vi "Check SUM.vi"() -> ()   [LabVIEW 2010, in "DCP551.lvlib"]
uses:
  DCP551.lvlib
panel:
  out "hex integer string 2":string
  out "Check Sum String":string
  in  "String Input":string
  out "*(type *) &x":string
  out "sum":u8 format="%04x"
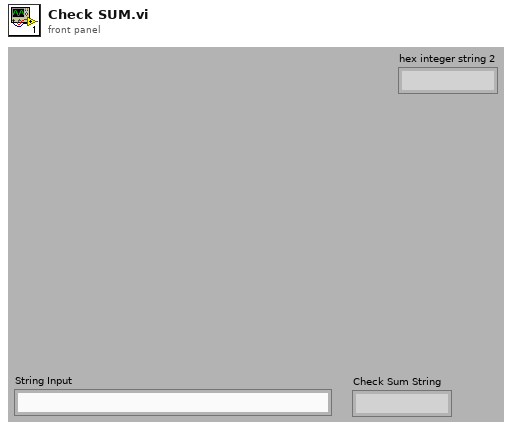
[diagram p1: front panel]
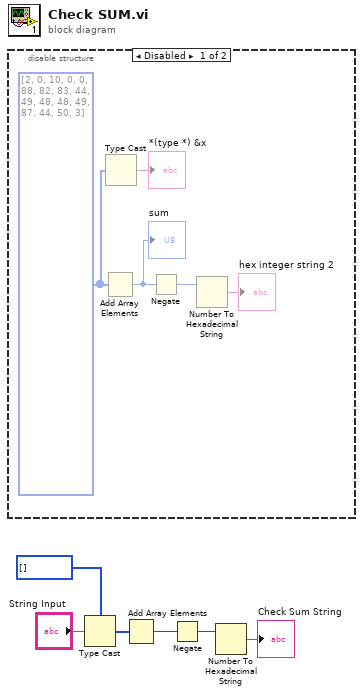
[diagram p0: block diagram]
diagram:
  n1 = disable-structure shown="Disabled" {
    frame Disabled {
      w11 = i8[] [2, 0, 10, 0, 0, 88, 82, 83, 44, 49, 48, 48, 49, 87, 44, 50, 3]
      n2 = Add Array Elements(numeric array=w11) -> (sum=w7:i8)
      "sum" <- w7
      n3 = Type Cast(x=w11) -> (*(type *) &x=→"*(type *) &x":string)  [unwired: 1 in]
      n4 = Negate(x=w7) -> (-x=w8:i8)
      n5 = Number To Hexadecimal String(2:w8) -> (0:→"hex integer string 2":string)  [unwired: 1 in]
    }
    frame Enabled {
    }
  }
  n6 = Type Cast(type=i8[] [], x="String Input") -> (*(type *) &x=w4:i8[])
  n7 = Add Array Elements(numeric array=w4) -> (sum=w3:i8)
  n8 = Negate(x=w3) -> (-x=w2:i8)
  n9 = Number To Hexadecimal String(2:w2) -> (0:→"Check Sum String":string)  [unwired: 1 in]
